vi "LVClass_CorrectionDataManager Compute_SlopesFromPositions.vi"(0 "CorrectionDataManager in":refnum<class "CorrectionDataManager.lvclass">, 5 "position":sgl[](array[numeric]), 7 "HasoSlopes in":refnum<class "HasoSlopes.lvclass">, 11 "error in (no error)":errorcluster) -> (4 "CorrectionDataManager out":refnum<class "CorrectionDataManager.lvclass">, 8 "HasoSlopes out":refnum<class "HasoSlopes.lvclass">, 15 "error out":errorcluster)   [LabVIEW 2020, in "CorrectionDataManager.lvclass"]
doc: "Simulation of the expected slopes given the Wavefront corrector preferences\nand an array of positions.\n\n--------------------------------------------------------------------------------\n\n<B>corrdata_managerIn </B> : CorrDataManager object.\n<B>corrdata_managerOut </B> : CorrDataManager object.\n<B>min </B> : WavefrontCorrector preferences : lowest command value.\n<B>max </B> : WavefrontCorrector preferences : highest command value.\n<B>validity </B> : WavefrontCorrector preferences : status.\n<B>fixed_values </B> : WavefrontCorrector preferences : fixed positions.\n<B>positions </B> : Array of size actuators count, containing for each actuator its current\n position.\n<B>HasoSlopes </B> : HasoSlopes object, where the simulated slopes are stored.\n<B>ErrorIn </B> : Error\n<B>ErrorOut </B> : Error\n\n--------------------------------------------------------------------------------"
uses:
  CorrectionDataManager.lvclass
  HasoSlopes.lvclass
  CorrectionDataManager.lvclass/CorrectionDataManager.ctl
  LVClass_HasoSlopes Read HasoSlopes _ property.vi
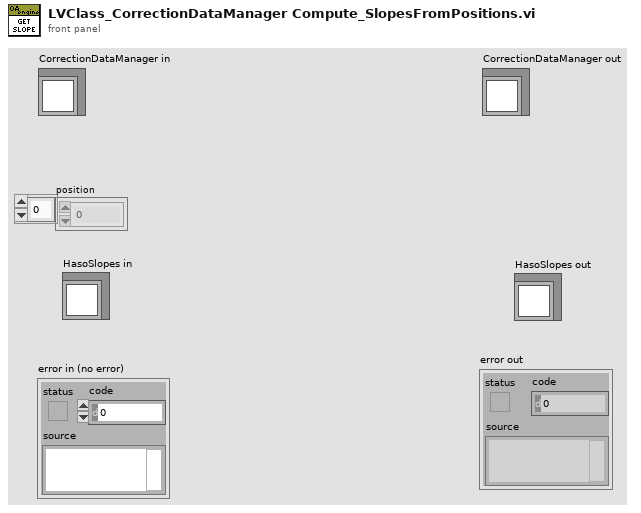
[diagram p1: front panel]
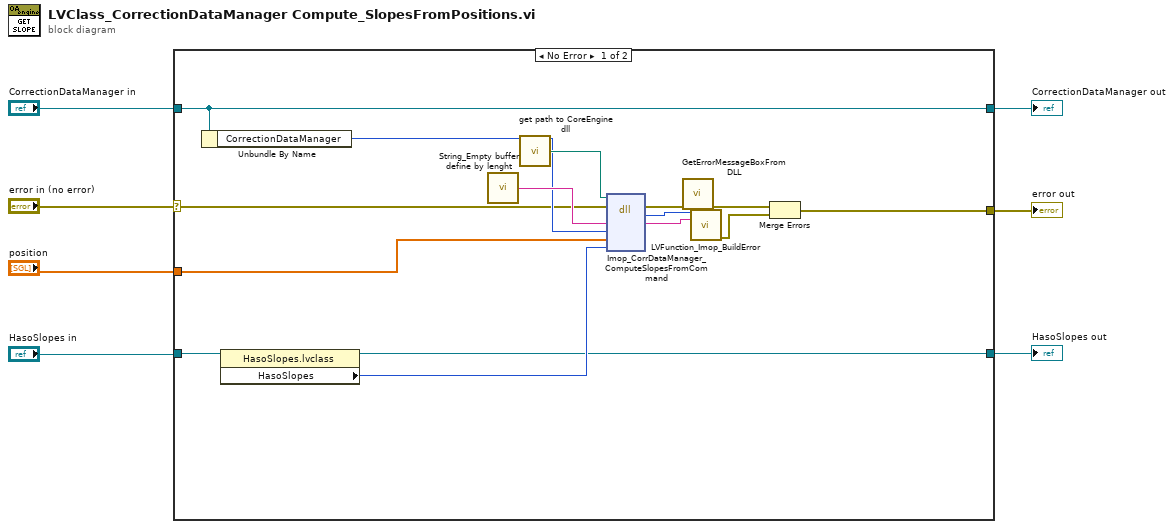
[diagram p0: block diagram]
diagram:
  n1 = case shown="No Error" "error in (no error)" {
    selector: "error in (no error)" -> [w10 w25]
    tunnel: [w20 w25] -> w5
    tunnel: [w19 w24] -> w4
    tunnel: "CorrectionDataManager in" -> [w19 w24]
    tunnel: "HasoSlopes in" -> [w12 w23]
    tunnel: [w9 w23] -> w2
    tunnel: "position" -> [w8 _]
    frame No Error {
      n2 = Unbundle By Name(w19) -> ("CorrectionDataManager"=w13:i32)
      n3 = property class="HasoSlopes.lvclass"(reference=w12) -> (reference out=w9:refnum<class "HasoSlopes.lvclass">, "HasoSlopes"=w11:i32)  [unwired: 1 in, 1 out]
      n4 = call "String_Empty buffer define by lenght.vi"() -> ("Empty buffer"=w17:string)  [unwired: 1 in]
      n5 = call "get path to CoreEngine dll.vi"() -> ("path to c_interface_vc100.dll"=w18:path)  [unwired: 12 in, 3 out]
      n6 = dll-call lib="D:/FLE/0.Code/CoreEngine4_Suite/LV2011_interface/DLLs/c_interface_vc100.dll" fn="Imop_CorrDataManager_ComputeSlopesFromCommand"(path in=w18, error in=w10, "message"=w17, "WavefrontCorrection"=w13, "position"=w8, "HasoSlopes"=w11) -> (error out=w16:errorcluster, "return type"=w15:i32, "message"=w14:string)  [unwired: 4 in, 1 out]
      n7 = call "GetErrorMessageBoxFromDLL.vi"("error IN"=w16) -> ("error OUT"=w22:errorcluster)  [unwired: 10 in]
      n8 = call "LVFunction_Imop_BuildError.vi"("code"=w15, "String to Prepend to source (\"\")"=w14) -> ("error out"=w21:errorcluster)  [unwired: 13 in]
      n9 = Merge Errors(w22, w21) -> (w20:errorcluster)
    }
    frame Error {
    }
  }
  "error out" <- w5
  "CorrectionDataManager out" <- w4
  "HasoSlopes out" <- w2
